vi "Debug_Report NB Records.vi"(8 "Decimation":i32, 9 "fill status":T2 items=["SEQ_EMPTY", "SEQ_PARTIAL", "SEQ_FULL"], 10 "run status":T1 items=["SEQ_STARTED", "SEQ_STOPPED", "SEQ_ERROR"], 11 "NB of Records Available":i32) -> ()   [LabVIEW 2020, in "Ballard Arinc-429 Engine.lvlib"]
uses:
  Ballard Arinc-429 Engine.lvlib
  <instrlib>/BTICardLib/Public/Controls/Seq Fill Status.ctl
  <instrlib>/BTICardLib/Public/Controls/Seq Run Status.ctl
  <vilib>/NI VeriStand/Custom Device Tools/Custom Device Utility Library/Custom Device Utility Library.lvlib
  <instrlib>/BTICardLib/BTICardLV.lvlib
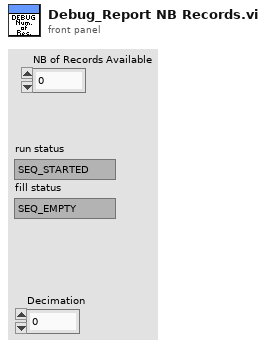
[diagram p1: front panel]
types:
  T1 = typedef "BTICardLV.lvlib/Seq Run Status.ctl" = u32
  T2 = typedef "BTICardLV.lvlib/Seq Fill Status.ctl" = u32
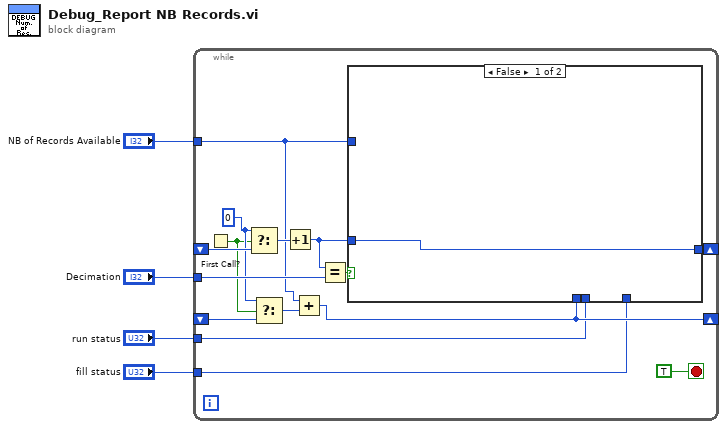
[diagram p0: block diagram]
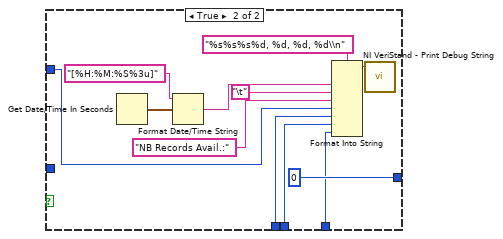
[diagram p2: hidden frame]
diagram:
  n1 = while {
    shift-right: [w13] -> _
    shift-left: _ -> [w16]
    tunnel: "Decimation" -> [w18]
    tunnel: "NB of Records Available" -> [w8]
    shift-right: [w7] -> _
    shift-left: _ -> [w10]
    tunnel: "run status" -> [w6]
    tunnel: "fill status" -> [w5]
    stop <- TRUE stop-if-true
    w12 = 0 ("Decimation")
    n2 = First Call?() -> (First Call?: T/F=w11:bool)
    n3 = Select(t=w12, s=w11, f=w16) -> (s? t:f=w15:i32)
    n4 = Select(t=w12, s=w11, f=w10) -> (s? t:f=w9:i32)
    n5 = Increment(x=w15) -> (x+1=w14:i32)
    n6 = Add(x=w8, y=w9) -> (x+y=w7:i32)
    n7 = Equal?(x=w14, y=w18) -> (x = y?=w17:bool)
    n8 = case shown="False" w17 {
      tunnel: w14 -> [w20 _]
      tunnel: [w20 0] -> w13
      tunnel: w8 -> [_ w24]
      tunnel: w7 -> [_ w23]
      tunnel: w6 -> [_ w21]
      tunnel: w5 -> [_ w22]
      frame False {
      }
      frame True {
        n9 = Get Date/Time In Seconds() -> (seconds since 1Jan1904=w31:timestamp)
        n10 = Format Date/Time String(time format string (%c)="[%H:%M:%S%3u]", seconds (now)=w31) -> (date/time string=w30:string)  [unwired: 1 in]
        n11 = Format Into String(format string="%s%s%s%d, %d, %d, %d\\n", w30, "\t", "NB Records Avail.:" ("initial string"), w24, w23, w21, w22) -> (resulting string=w29:string)  [unwired: 2 in, 1 out]
        n12 = call <vilib>:"NI VeriStand - Print Debug String.vi"("Message"=w29) -> ()  [unwired: 10 in, 1 out]
      }
    }
  }
